vi "F020_ain_get.vi"(8 "error in":errorcluster, 10 "Cluster":T1={"ADDRESS[0.255]"=170, "AIN CHANNEL[0..7]"=0, "gain"=0}, 11 "COM in":string="COM4") -> (0 "error out":errorcluster={"status"=TRUE, "code"=-1073807343, "source"=""}, 2 "ain":sgl format="%.2f", 3 "COM out":string="COM4")   [LabVIEW 2016]
doc: "This example performs a serial port write and a serial port read. The parameters set for the serial port must match the parameters of the connected instrument or device. The VISA Configure Serial Port VI sets the configuration parameters. The front panel displays the controls used to configure the basic parameters, such as baud rate, data bits, and parity. The VI passes the VISA resource name to other VIs that perform operations on that VISA resource. The VISA Write function sends a command to the serial device and the VISA Read function returns data based on the command. The VISA Close function then closes the reference to the serial device. It is important to close the reference; otherwise, further communication through that port might not be possible."
panel:
  out "return count":u32
  out "packet ( <xxAABBCC..>":string="<03AA1301>"
  out "Response {xxxx...}":string
  # "loopback: <xxAABB>\nwr_dout:   <xxAA11aabbccdd> aa=ch, bb=val, ccdd=timeout[sec]\nrd_ain:      <xxAA13aa> -> {qqww}"
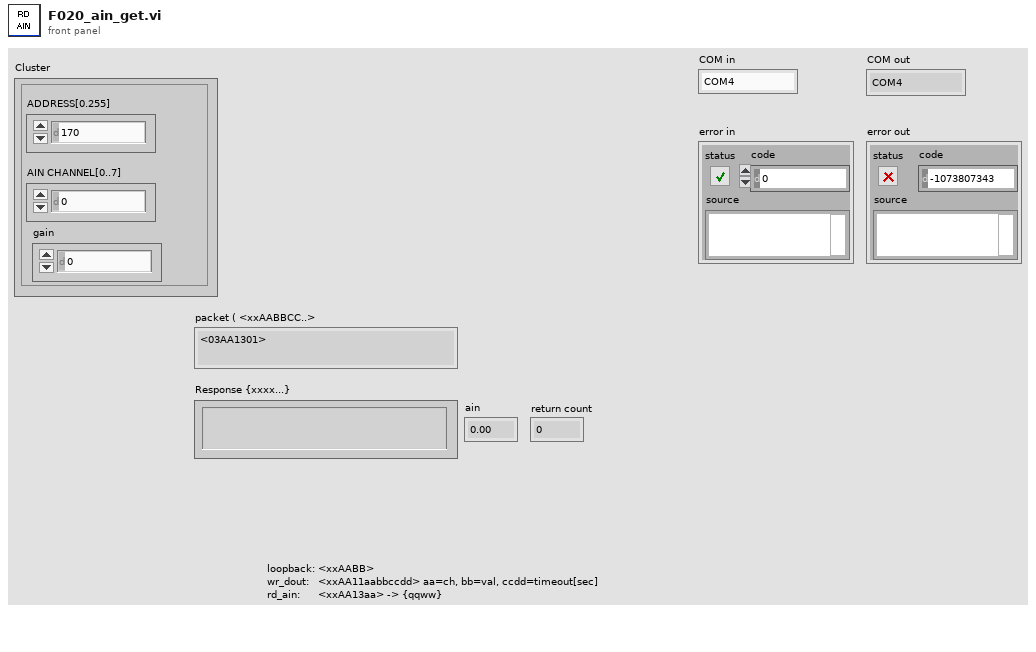
[diagram p1: front panel]
types:
  T1 = cluster{"ADDRESS[0.255]":u8, "AIN CHANNEL[0..7]":u8, "gain":u8}
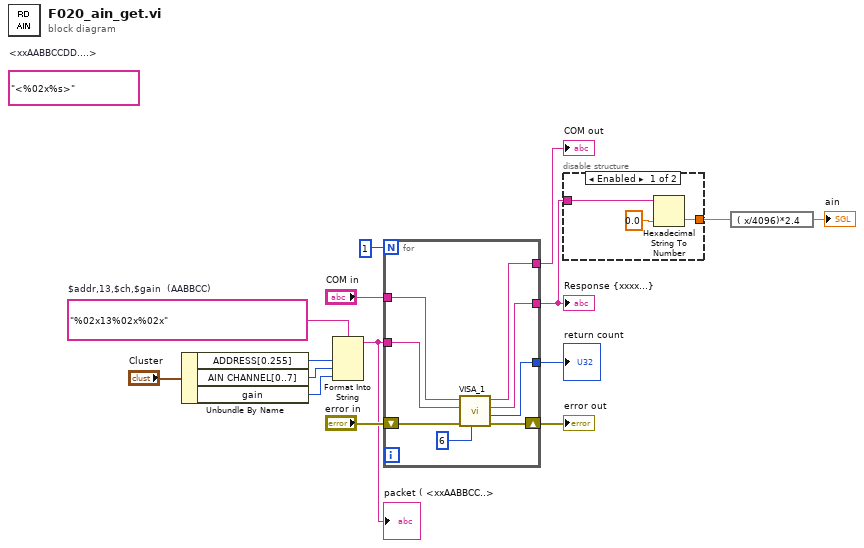
[diagram p0: block diagram]
diagram:
  (unwired) "<%02x%s>"  # <xxAABBCCDD....>
  w11 = "%02x13%02x%02x"  # $addr,13,$ch,$gain  (AABBCC)
  n1 = Unbundle By Name("Cluster") -> ("ADDRESS[0.255]"=w9:u8, "AIN CHANNEL[0..7]"=w7:u8, "gain"=w3:u8)
  n2 = Format Into String(format string=w11, w9, w7, w3) -> (resulting string=w6:string)  [unwired: 2 in, 1 out]
  "packet ( <xxAABBCC..>" <- w6
  n3 = for {
    N: 1 -> [_]
    shift-right: [w18] -> w5
    shift-left: "error in" -> [w20]
    tunnel: "COM in" -> [w23]
    tunnel: [w22] -> w15
    tunnel: w6 -> [w21]
    tunnel: [w17] -> w12
    tunnel: [w16] -> w1
    n4 = call "VISA_1.vi"("delay[ms]"=u32 6, "error in"=w20, "wr_buf"=w21, "COM in"=w23) -> ("error out"=w18:errorcluster, "return count"=w16:u32, "rx_buf"=w17:string, "COM out"=w22:string)  [unwired: 4 in]
  }
  "Response {xxxx...}" <- w12
  "error out" <- w5
  "return count" <- w1
  "COM out" <- w15
  n5 = disable-structure shown="Enabled" {
    disable-tunnel: w12 -> [w24 _]
    disable-tunnel: [w25 _] -> w8
    frame Enabled {
      n6 = Hexadecimal String To Number(string=w24, default (0uL)=sgl 0.0 ("default (0 U32)")) -> (number=w25:sgl)  [unwired: 1 in, 1 out]
    }
    frame Disabled {
    }
  }
  n7 = expression code="( x/4096)*2.4"(w8) -> (→"ain":sgl)
